vi "Measurement UI.vi"() -> ()   [LabVIEW 2025, in "FGEN Arb Sequence Mode UI.lvlib"]
uses:
  FGEN Arb Sequence Mode UI.lvlib
  508e06a4-d1fa-4daf-8eae-7928ac733f97.vi
  84f7658a-f4d0-49fe-a9b6-8e25366cdade.vi
panel:
  in  "More":bool
  out "FGEN Sample Rate":dbl format="%#_6pHz"
  in  "Markers Sequence":i32[](array[numeric])
  in  "Loops Sequence":u32[](array[numeric])
  in  "Waveform Sequence (Cluster)":T1(array[cluster])=[{"Wfm"="Wfm1", "Loops"=1, "Marker"=0}] caption="Waveform Sequence"
  in  "Waveform Sequence":string[](array[string])
  in  "TDMS File Path":path
  in  "TDMS Name Mapping":enum32{"Channels", "Groups"}(tab)
  in  "TDMS Channels":string[](array[combo])
  in  "FGEN Resource Names":string[](array[combo])
  in  "Auto Name Wfm":bool
  in  "TDMS Groups":string[](array[combo])
  in  "FGEN Waveform Names":string[](array[string])=["Wfm1"] caption="FGEN Wfm Names"
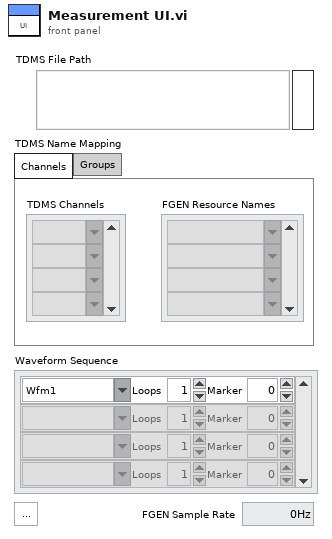
[diagram p1: front panel]
types:
  T1 = cluster{"Wfm":string, "Loops":u32, "Marker":i32}[]
  T2 = cluster{"TDMS Channels 2":string, "Loops":u32, "Loops":i32}
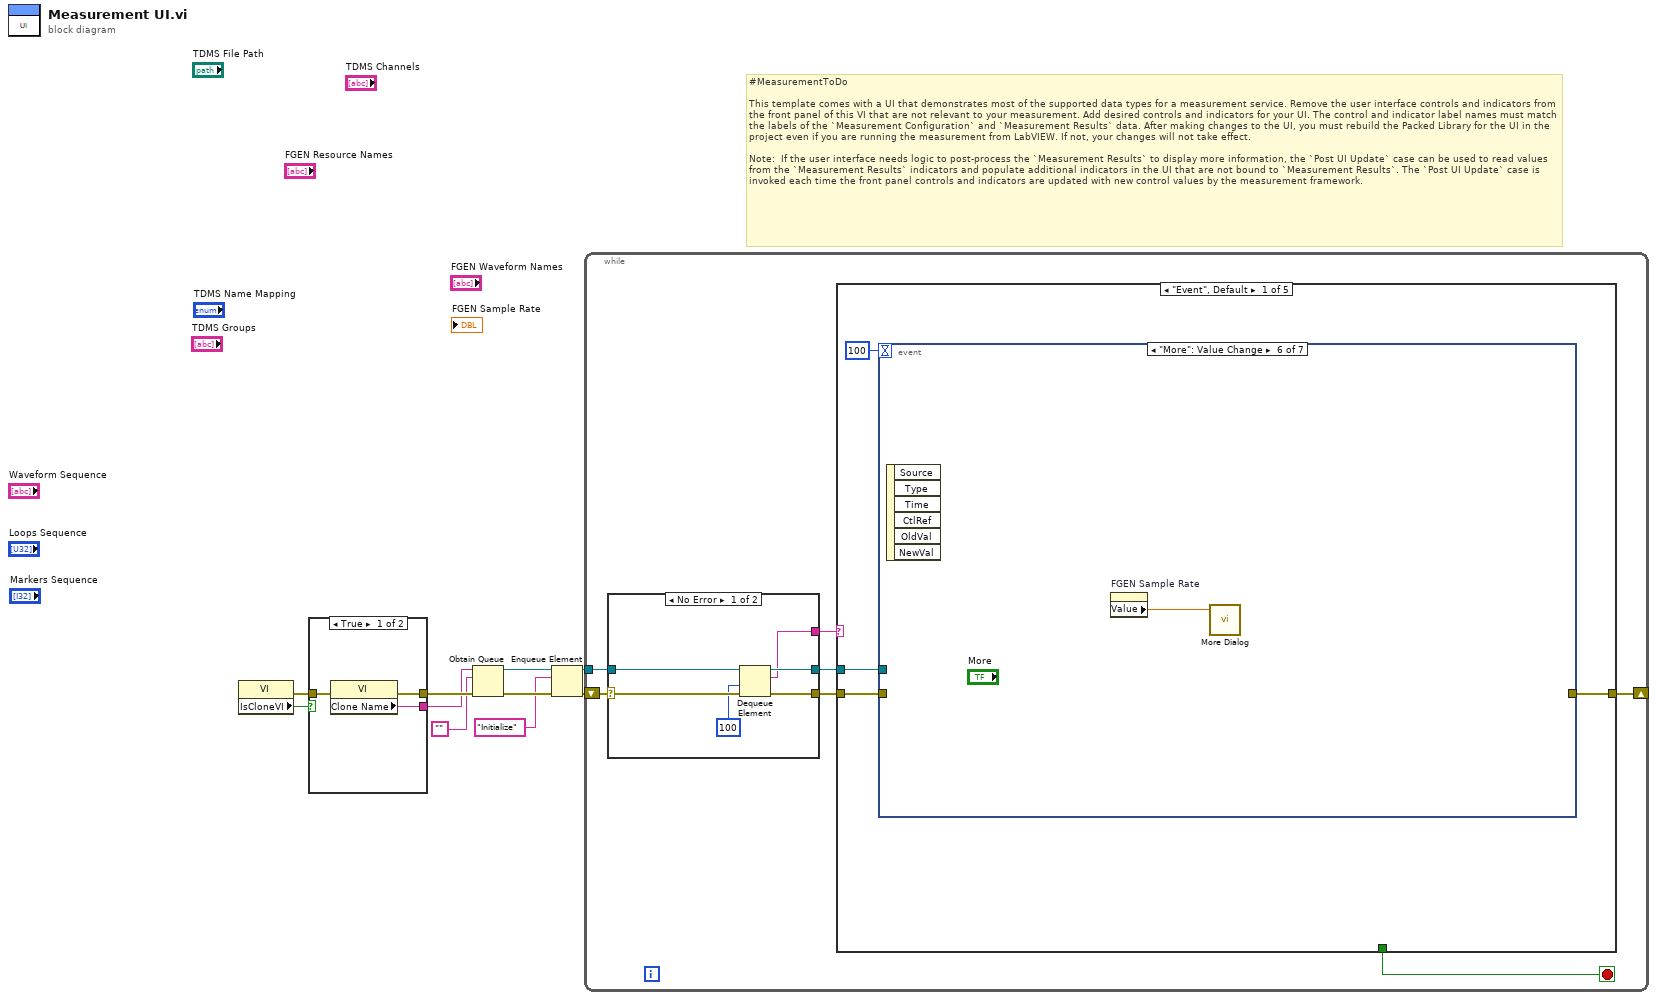
[diagram p0: block diagram]
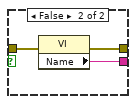
[diagram p2: hidden frame]
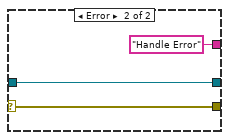
[diagram p3: hidden frame]
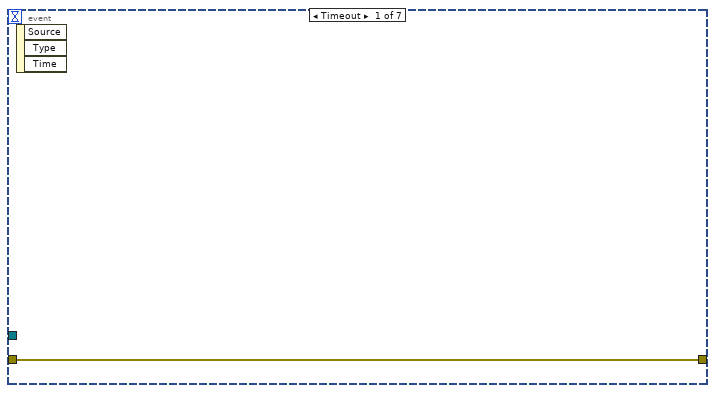
[diagram p4: hidden frame]
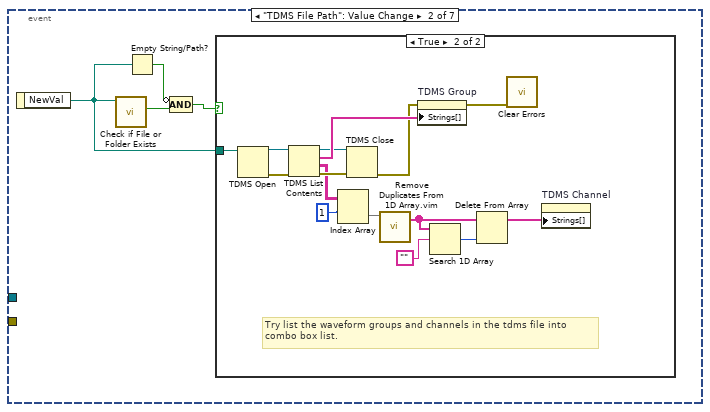
[diagram p5: hidden frame]
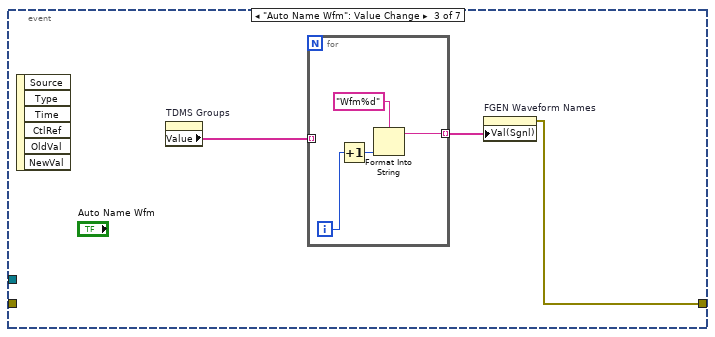
[diagram p7: hidden frame]
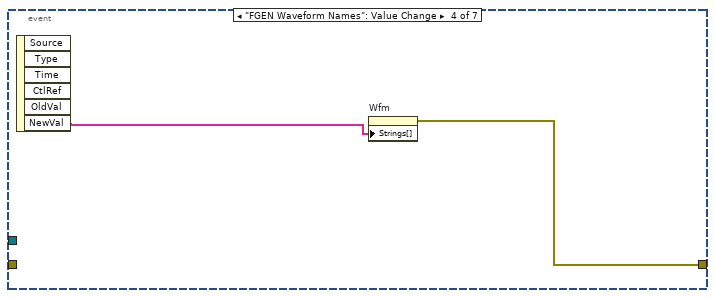
[diagram p8: hidden frame]
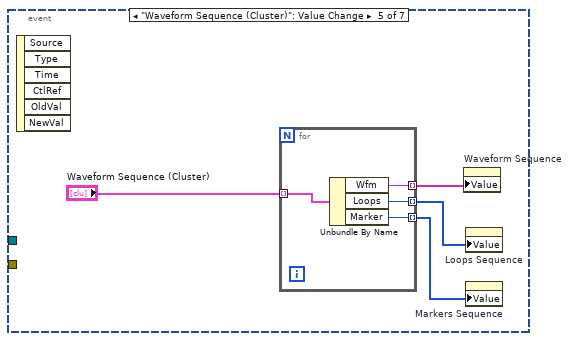
[diagram p9: hidden frame]
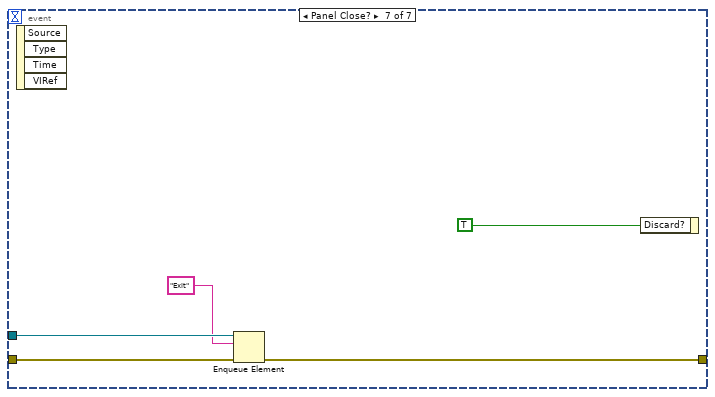
[diagram p10: hidden frame]
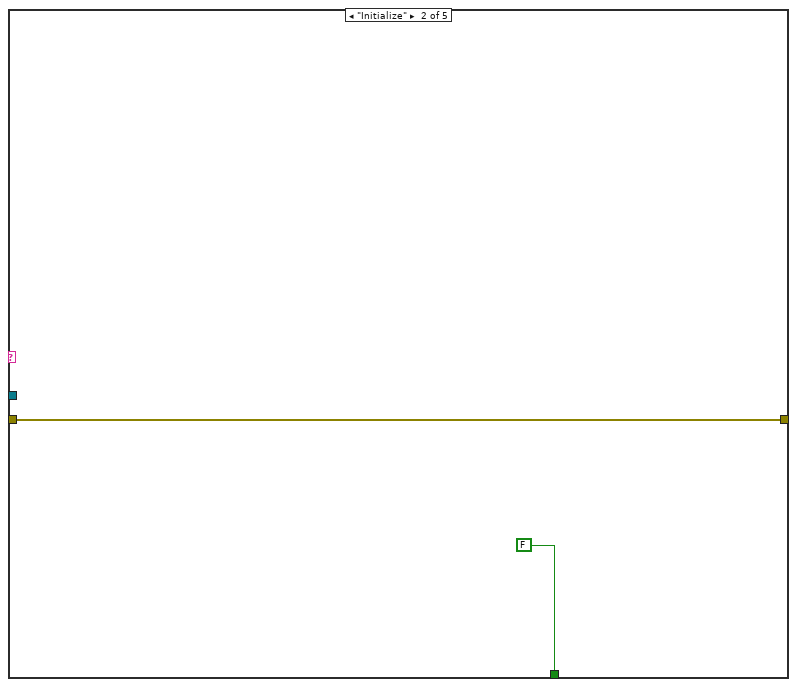
[diagram p11: hidden frame]
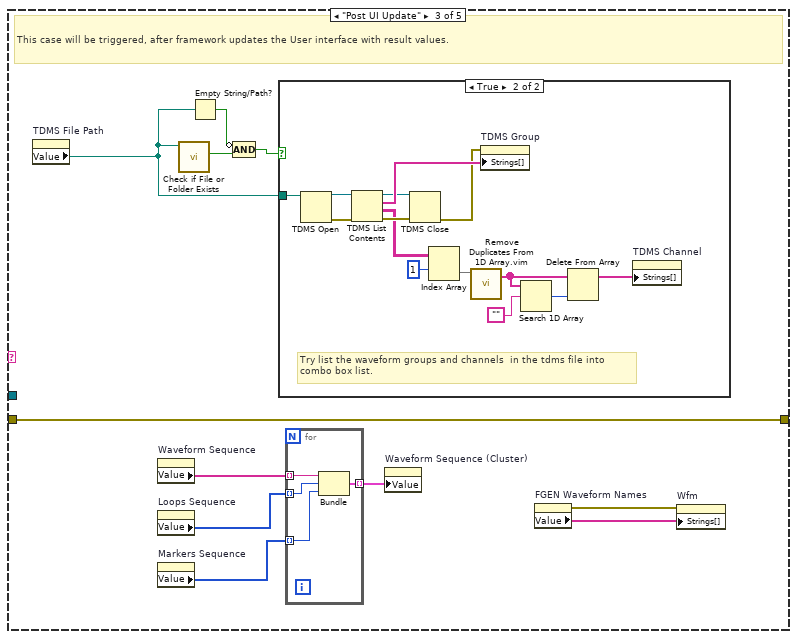
[diagram p12: hidden frame]
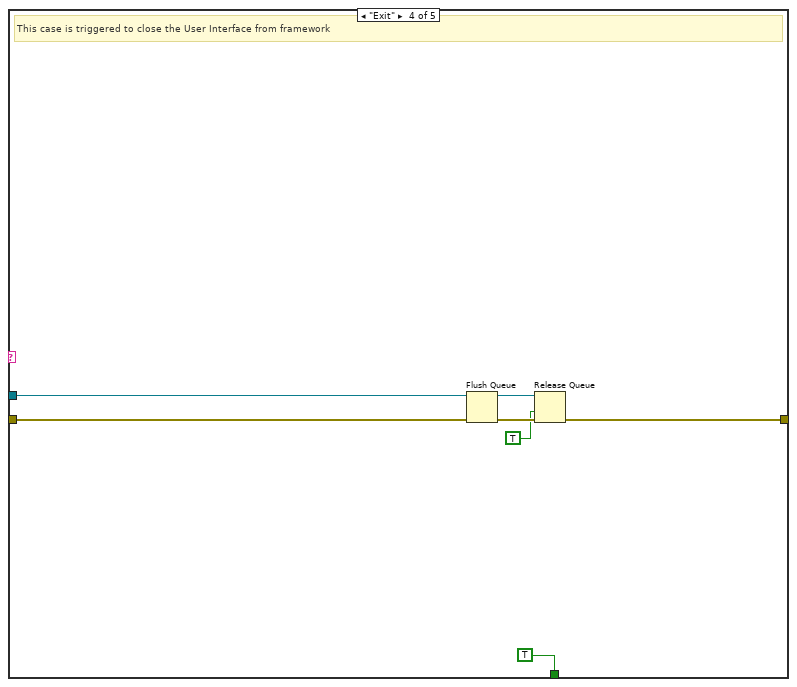
[diagram p14: hidden frame]
diagram:
  # "#MeasurementToDo  \n\nThis template comes with a UI that demonstrates most of the supported data types for a measurement service. Remove the user interface controls and indicators from the front panel of this VI that are not relevant to your measurement. Add desired controls and indicators for your UI. The control and indicator label names must match the labels of the `Measurement Configuration` and `Measurement Results` data. After making changes to the UI, you must rebuild the Packed Library for the UI in the project even if you are running the measurement from LabVIEW. If not, your changes will not take effect.\n\nNote:  If the user interface needs logic to post-process the `Measurement Results` to display more information, the `Post UI Update` case can be used to read values from the `Measurement Results` indicators and populate additional indicators in the UI that are not bound to `Measurement Results`. The `Post UI Update` case is invoked each time the front panel controls and indicators are updated with new control values by the measurement framework."
  n1 = property class="VI"() -> (error out=w1:errorcluster, "IsCloneVI"=w2:bool)  [unwired: 2 in, 1 out]
  n2 = case shown="True" w2 {
    tunnel: [w13 w16] -> w10
    tunnel: [w12 w15] -> w9
    tunnel: w1 -> [w11 w14]
    frame True {
      n3 = property class="VI"(error in=w11) -> (error out=w13:errorcluster, "Clone Name"=w12:string)  [unwired: 1 in, 1 out]
    }
    frame False {
      n4 = property class="VI"(error in=w14) -> (error out=w16:errorcluster, "Name"=w15:string)  [unwired: 1 in, 1 out]
    }
  }
  n5 = Obtain Queue(name (unnamed)=w9, element data type="", error in (no error)=w10) -> (queue out=w6:refnum<queue>, error out=w8:errorcluster)  [unwired: 2 in, 1 out]
  n6 = Enqueue Element(queue=w6, element="Initialize", error in (no error)=w8) -> (queue out=w5:refnum<queue>, error out=w7:errorcluster)  [unwired: 1 in, 1 out]
  n7 = while {
    shift-right: [w17] -> _
    shift-left: w7 -> [w23]
    tunnel: w5 -> [w21]
    stop <- w18 stop-if-true
    n8 = case shown="No Error" w23 {
      selector: w23 -> [w29 w32]
      tunnel: [w28 w32] -> w22
      tunnel: w21 -> [w27 w31]
      tunnel: [w26 w31] -> w20
      tunnel: [w25 "Handle Error"] -> w19
      frame No Error {
        n9 = Dequeue Element(queue=w27, timeout in ms (-1)=100, error in (no error)=w29) -> (queue out=w26:refnum<queue>, element=w25:string, error out=w28:errorcluster)  [unwired: 1 out]
      }
      frame Error {
      }
    }
    n10 = case shown="\"Event\", Default" w19 {
      tunnel: w22 -> [w35 w81 w92 w117 w118]
      tunnel: w20 -> [w33 _ _ w115 _]
      tunnel: [w36 w81 w92 w112 w118] -> w17
      tunnel: [_ FALSE _ TRUE _] -> w18
      frame "Event", Default {
        n11 = event shown="[5] \"More\": Value Change" {
          selector: _ -> [_ _ _ _ _ _ _]
          dyn-events: _ -> [_ _ _ _ _ _ _]
          timeout: 100 -> [_ _ _ _ _ _ _]
          tunnel: [w37 _ w57 w65 _ _ w77] -> w36
          tunnel: w35 -> [w37 _ _ _ _ _ w78]
          tunnel: w33 -> [_ _ _ _ _ _ w76]
          event Timeout {
            n12 = event-data() -> ()  [unwired: 1 in, 3 out]
          }
          event "TDMS File Path": Value Change {
            n13 = event-data() -> ("NewVal"=w38:path)  [unwired: 1 in]
            n14 = call <vilib>:"Check if File or Folder Exists.vi"("path"=w38) -> ("file or folder exists?"=w41:bool)  [unwired: 8 in, 2 out]
            n15 = Empty String/Path?(string/path=w38) -> (empty?=w39:bool)
            n16 = Compound Arithmetic op=AND(invert w39, w41) -> (w40:bool)
            n17 = case shown="True" w40 {
              tunnel: w38 -> [_ w56]
              frame False {
              }
              frame True {
                # "Try list the waveform groups and channels in the tdms file into \ncombo box list."
                n18 = TDMS Open(11:w56) -> (0:w51:errorcluster, 3:w55:refnum<k34>)  [unwired: 6 in]
                n19 = TDMS List Contents(4:w51, 7:w55) -> (0:w53:errorcluster, 1:w48:string[][], 2:w54:string[], 3:w52:refnum<k34>)  [unwired: 1 in]
                n20 = Index Array(array=w48, index (row)=1) -> (element=w46:string[])  [unwired: 1 in]
                n21 = TDMS Close(8:w53, 11:w52) -> (0:w50:errorcluster)  [unwired: 1 out]
                n22 = call "Remove Duplicates From 1D Array.vim"("array"=w46) -> ("array with duplicates removed"=w43:string[])  [unwired: 10 in]
                n23 = property on="TDMS Group" class="CmbBox"(error in=w50, "Strings[]"=w54) -> (error out=w49:errorcluster)  [unwired: 1 in, 1 out]
                n24 = Search 1D Array(1D array=w43, element="") -> (index of element=w44:i32)  [unwired: 1 in]
                n25 = Delete From Array(array=w43, index=w44) -> (array with subset deleted=w42:string[])  [unwired: 1 in, 1 out]
                n26 = call <vilib>:"Clear Errors.vi"("error in (no error)"=w49) -> ()  [unwired: 5 in, 2 out]
                n27 = property on="TDMS Channel" class="CmbBox"("Strings[]"=w42) -> ()  [unwired: 2 in, 2 out]
              }
            }
          }
          event "Auto Name Wfm": Value Change {
            n28 = event-data() -> ()  [unwired: 1 in, 6 out]
            n29 = property on="TDMS Groups" class="Arr (strict)"() -> ("Value"=w59:string[])  [unwired: 2 in, 2 out]
            n30 = for {
              tunnel: w59 -> [_] mode=indexing
              tunnel: [w60] -> w58 mode=indexing
              i -> [w61]
              n31 = Increment(x=w61) -> (x+1=w62:i32)
              n32 = Format Into String(format string="Wfm%d", w62) -> (resulting string=w60:string)  [unwired: 2 in, 1 out]
            }
            n33 = property on="FGEN Waveform Names" class="Arr (strict)"("Val(Sgnl)"=w58) -> (error out=w57:errorcluster)  [unwired: 2 in, 1 out]
          }
          event "FGEN Waveform Names": Value Change {
            n34 = event-data() -> ("NewVal"=w64:string[])  [unwired: 1 in, 5 out]
            n35 = property on="Wfm" class="CmbBox"("Strings[]"=w64) -> (error out=w65:errorcluster)  [unwired: 2 in, 1 out]
          }
          event "Waveform Sequence (Cluster)": Value Change {
            n36 = event-data() -> ()  [unwired: 1 in, 6 out]
            n37 = for {
              tunnel: "Waveform Sequence (Cluster)" -> [w73] mode=indexing
              tunnel: [w72] -> w68 mode=indexing
              tunnel: [w71] -> w67 mode=indexing
              tunnel: [w70] -> w66 mode=indexing
              n38 = Unbundle By Name(w73) -> ("Wfm"=w72:string, "Loops"=w71:u32, "Marker"=w70:i32)
            }
            n39 = property on="Waveform Sequence" class="Arr (strict)"("Value"=w68) -> ()  [unwired: 2 in, 2 out]
            n40 = property on="Loops Sequence" class="Arr (strict)"("Value"=w67) -> ()  [unwired: 2 in, 2 out]
            n41 = property on="Markers Sequence" class="Arr (strict)"("Value"=w66) -> ()  [unwired: 2 in, 2 out]
          }
          event "More": Value Change {
            n42 = event-data() -> ()  [unwired: 1 in, 6 out]
            n43 = property on="FGEN Sample Rate" class="DigNum (strict)"() -> ("Value"=w74:dbl)  [unwired: 2 in, 2 out]
            n44 = call "More Dialog.vi"("FGEN Sample Rate (Reference)"=w74) -> ()  [unwired: 11 in]
          }
          event Panel Close? {
            n45 = event-data() -> ()  [unwired: 1 in, 4 out]
            n46 = Enqueue Element(queue=w76, element="Exit", error in (no error)=w78) -> (error out=w77:errorcluster)  [unwired: 1 in, 2 out]
            n47 = event-data("Discard?"=TRUE) -> ()  [unwired: 1 in, 1 out]
          }
        }
      }
      frame "Initialize" {
      }
      frame "Post UI Update" {
        # "This case will be triggered, after framework updates the User interface with result values."
        n48 = property on="TDMS File Path" class="Path"() -> ("Value"=w88:path)  [unwired: 2 in, 2 out]
        n49 = property on="Waveform Sequence" class="Arr (strict)"() -> ("Value"=w87:string[])  [unwired: 2 in, 2 out]
        n50 = property on="Loops Sequence" class="Arr (strict)"() -> ("Value"=w86:u32[])  [unwired: 2 in, 2 out]
        n51 = property on="Markers Sequence" class="Arr (strict)"() -> ("Value"=w82:i32[])  [unwired: 2 in, 2 out]
        n52 = call <vilib>:"Check if File or Folder Exists.vi"("path"=w88) -> ("file or folder exists?"=w91:bool)  [unwired: 8 in, 2 out]
        n53 = Empty String/Path?(string/path=w88) -> (empty?=w89:bool)
        n54 = Compound Arithmetic op=AND(invert w89, w91) -> (w90:bool)
        n55 = case shown="True" w90 {
          tunnel: w88 -> [_ w110]
          frame False {
          }
          frame True {
            # "Try list the waveform groups and channels  in the tdms file into \ncombo box list."
            n56 = TDMS Open(11:w110) -> (0:w105:errorcluster, 3:w109:refnum<k34>)  [unwired: 6 in]
            n57 = TDMS List Contents(4:w105, 7:w109) -> (0:w107:errorcluster, 1:w97:string[][], 2:w108:string[], 3:w106:refnum<k34>)  [unwired: 1 in]
            n58 = TDMS Close(8:w107, 11:w106) -> (0:w104:errorcluster)  [unwired: 1 out]
            n59 = Index Array(array=w97, index (row)=1) -> (element=w103:string[])  [unwired: 1 in]
            n60 = call "Remove Duplicates From 1D Array.vim"("array"=w103) -> ("array with duplicates removed"=w101:string[])  [unwired: 10 in]
            n61 = property on="TDMS Group" class="CmbBox"(error in=w104, "Strings[]"=w108) -> ()  [unwired: 1 in, 2 out]
            n62 = Search 1D Array(1D array=w101, element="") -> (index of element=w102:i32)  [unwired: 1 in]
            n63 = Delete From Array(array=w101, index=w102) -> (array with subset deleted=w100:string[])  [unwired: 1 in, 1 out]
            n64 = property on="TDMS Channel" class="CmbBox"("Strings[]"=w100) -> ()  [unwired: 2 in, 2 out]
          }
        }
        n65 = for {
          tunnel: w87 -> [w96] mode=indexing
          tunnel: w86 -> [w95] mode=indexing
          tunnel: [w94] -> w85 mode=indexing
          tunnel: w82 -> [w93] mode=indexing
          n66 = Bundle("TDMS Channels 2"=w96, "Loops"=w95, "Loops"=w93) -> (w94:T2)  [unwired: 1 in]
        }
        n67 = property on="Waveform Sequence (Cluster)" class="Arr (strict)"("Value"=w85) -> ()  [unwired: 2 in, 2 out]
        n68 = property on="FGEN Waveform Names" class="Arr (strict)"() -> (error out=w83:errorcluster, "Value"=w84:string[])  [unwired: 2 in, 1 out]
        n69 = property on="Wfm" class="CmbBox"(error in=w83, "Strings[]"=w84) -> ()  [unwired: 1 in, 2 out]
      }
      frame "Exit" {
        # "This case is triggered to close the User Interface from framework"
        n70 = Flush Queue(queue=w115, error in (no error)=w117) -> (queue out=w114:refnum<queue>, error out=w113:errorcluster)  [unwired: 1 out]
        n71 = Release Queue(queue=w114, force destroy? (F)=TRUE, error in (no error)=w113) -> (error out=w112:errorcluster)  [unwired: 2 out]
      }
      frame "Handle Error" {
      }
    }
  }
